vi "ep_Check Window Length.vi"(8 "error in (no error)":errorcluster, 11 "window length [s]":dbl) -> (0 "error out":errorcluster)   [LabVIEW 2014, in "NI_EP_Motor Monitoring.lvlib"]
uses:
  <vilib>/addons/Electrical Power/Motor Monitoring/NI_EP_Motor Monitoring.lvlib
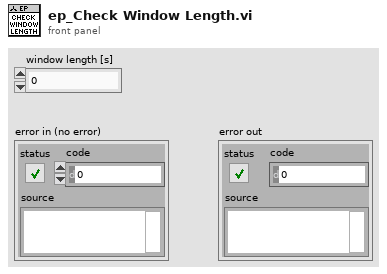
[diagram p1: front panel]
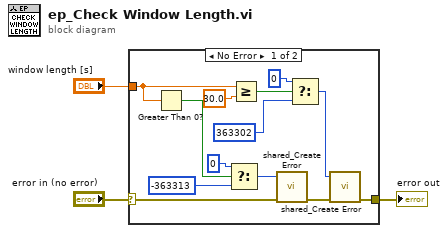
[diagram p0: block diagram]
diagram:
  n1 = case shown="No Error" "error in (no error)" {
    selector: "error in (no error)" -> [w12 w17]
    tunnel: [w4 w17] -> w2
    tunnel: "window length [s]" -> [w5 _]
    frame No Error {
      n2 = Greater Than 0?(x=w5) -> (x > 0?=w16:bool)
      n3 = Select(t=0 ("error code (0)"), s=w16, f=-363313 ("error code (0)")) -> (s? t:f=w13:i32)
      n4 = Greater Or Equal?(x=w5, y=30.0) -> (x >= y?=w10:bool)
      n5 = call <vilib>:"shared_Create Error.vi"("error in (no error)"=w12, "error code (0)"=w13) -> ("error out"=w7:errorcluster)  [unwired: 9 in]
      n6 = Select(t=0 ("error code (0)"), s=w10, f=363302) -> (s? t:f=w6:i32)
      n7 = call <vilib>:"shared_Create Error.vi"("error in (no error)"=w7, "error code (0)"=w6) -> ("error out"=w4:errorcluster)  [unwired: 9 in]
    }
    frame Error {
    }
  }
  "error out" <- w2
